vi "List Tests.vi"(8 "error in (no error)":errorcluster, 11 "LUnit Test Suite In":refnum<class "LUnit Test Suite.lvclass">) -> (0 "error out":errorcluster, 2 "Tests":string[](array[string]), 3 "LUnit Test Suite Out":refnum<class "LUnit Test Suite.lvclass">)   [LabVIEW 2020, in "LUnit Test Suite.lvclass"]
uses:
  LUnit Test Suite.lvclass
  LUnit Test Suite.lvclass/LUnit Test Suite.ctl
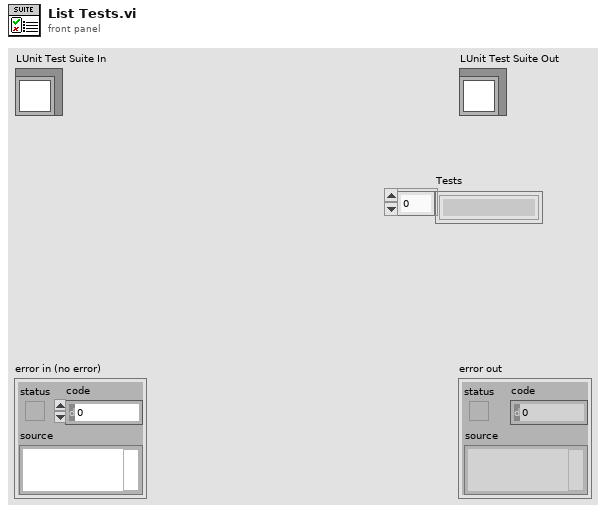
[diagram p1: front panel]
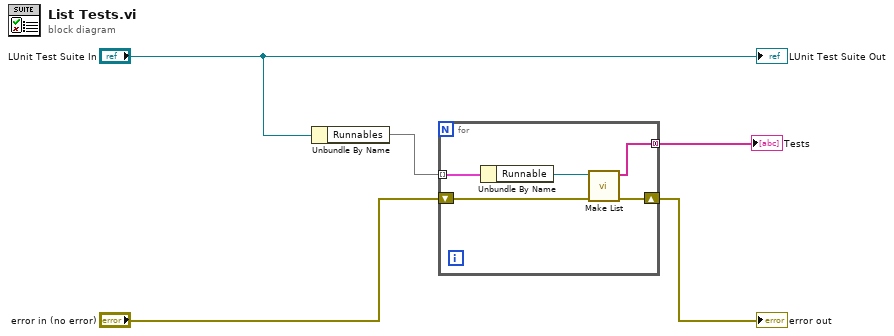
[diagram p0: block diagram]
diagram:
  n1 = Unbundle By Name("LUnit Test Suite In") -> ("Runnables"=w4:map{string, refnum<class "Runnable.lvclass">})
  n2 = for {
    tunnel: w4 -> [w10] mode=indexing
    tunnel: [w8] -> w3 mode=concatenating
    shift-right: [w7] -> w2
    shift-left: "error in (no error)" -> [w6]
    n3 = Unbundle By Name(w10) -> ("Runnable"=w9:refnum<class "Runnable.lvclass">)
    n4 = call "Make List.vi"("error in (no error)"=w6, "Runnable in"=w9) -> ("error out"=w7:errorcluster, "List of Runnables"=w8:string[])  [unwired: 8 in]
  }
  "error out" <- w2
  "Tests" <- w3
  "LUnit Test Suite Out" <- "LUnit Test Suite In"
